vi "check_try_find_session.vi"(6 "main_db_path":path, 7 "Sesions":T1) -> (3 "SessionOut":T1)   [LabVIEW 2011]
panel:
  out "dup path":path
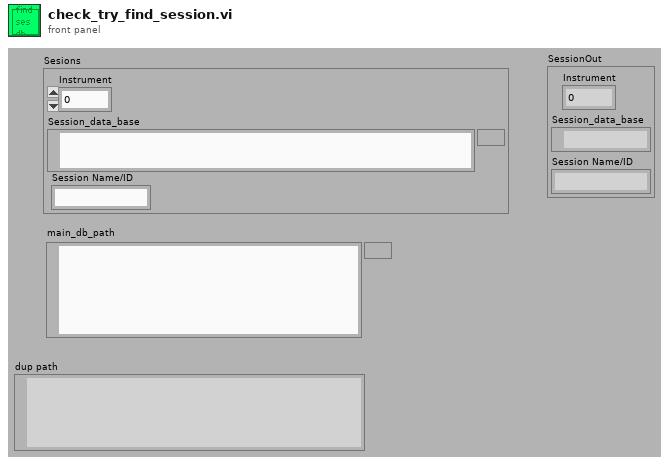
[diagram p1: front panel]
types:
  T1 = cluster{"Instrument":u16, "Session_data_base":path, "Session Name/ID":string}
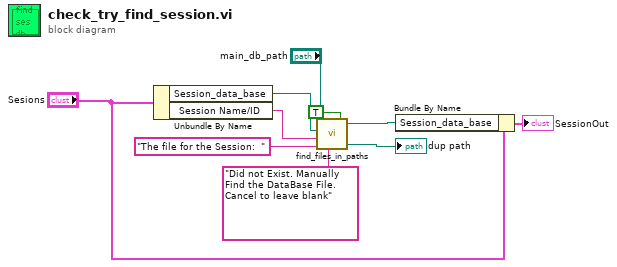
[diagram p0: block diagram]
diagram:
  n1 = Unbundle By Name("Sesions") -> ("Session_data_base"=w10:path, "Session Name/ID"=w9:string)
  n2 = call "find_files_in_paths.vi"("TopLevelDataFilePath"="main_db_path", "File2Find"=w10, "Item Name"=w9, "Message Prefix"="The file for the Session:  " ("prompt"), "What to do string/file prompt"="Did not Exist. Manually Find the DataBase File. Cancel to leave blank" ("string"), "PromptFormissingFile"=TRUE) -> ("Path"=w4:path, "Relative Path to file"=→"dup path":path)
  n3 = Bundle By Name(cluster="Sesions", "Session_data_base"=w4) -> (→"SessionOut":T1)
